vi "Handler Launch Failure.vi"(8 "error in (no error)":errorcluster) -> (0 "error out":errorcluster)   [LabVIEW 2013, in "Modbus Library - Advance.lvlib" / "TCP Slave.lvclass"]
doc: "Displays a message which lets the user know that an error has occured when launching the slave."
uses:
  TCP Slave.lvclass
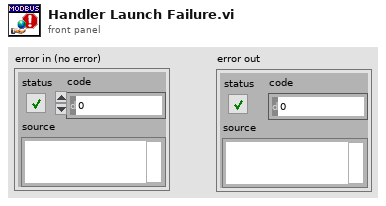
[diagram p1: front panel]
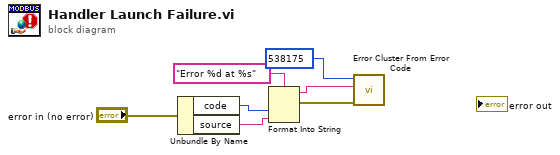
[diagram p0: block diagram]
diagram:
  n1 = Unbundle By Name("error in (no error)") -> ("code"=w4:i32, "source"=w5:string)
  n2 = Format Into String(format string="Error %d at %s", w4, w5) -> (resulting string=w2:string, error out=w6:errorcluster)  [unwired: 2 in]
  n3 = call <vilib>:"Error Cluster From Error Code.vi"("error in (no error)"=w6, "error message (\"\")"=w2, "error code (0)"=538175) -> ()  [unwired: 6 in, 1 out]
